vi "Generate Subclasses.vi"(8 "Class Ref Map":T1, 9 "Owning LVLib":refnum<vi>, 10 "Inheritance Map":T1, 11 "Base Class":refnum<vi>) -> (0 "Augmented Class Ref Map":T1, 1 "Owning LVLib Dup":refnum<vi>, 2 "Reduced Inheritance Map":T1, 3 "Base Class Dup":refnum<vi>)   [LabVIEW 2013]
uses:
  <userlib>/ICON Technologies/ICON Maps/lvlib/Map.ctl
  <userlib>/ICON Technologies/ICON Maps/ICON Maps.lvlib
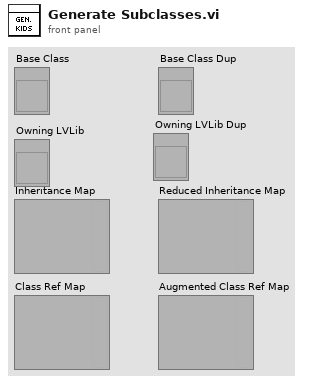
[diagram p1: front panel]
types:
  T1 = typedef "ICON Maps.lvlib/Map.ctl" = variant
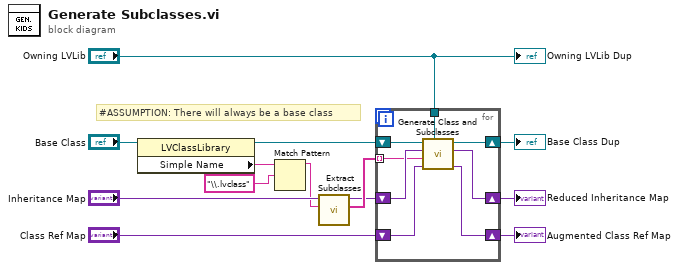
[diagram p0: block diagram]
diagram:
  # "#ASSUMPTION: There will always be a base class"
  n1 = property class="LVClassLibrary"(reference="Base Class") -> (reference out=w4:refnum<vi>, "Simple Name"=w7:string)  [unwired: 1 in, 1 out]
  n2 = Match Pattern(string=w7, regular expression="\\.lvclass") -> (before substring=w6:string)  [unwired: 1 in, 3 out]
  n3 = call "Extract Subclasses.vi"("Base Class Name"=w6, "Inheritance Map"="Inheritance Map") -> ("Subclass Names"=w12:string[], "Reduced Inheritance Map"=w11:T1)  [unwired: 8 in]
  n4 = for {
    tunnel: "Owning LVLib" -> [w21]
    tunnel: w12 -> [w18] mode=indexing
    shift-right: [w20] -> w9
    shift-left: w11 -> [w19]
    shift-right: [w16] -> w13
    shift-left: w4 -> [w17]
    shift-right: [w14] -> w1
    shift-left: "Class Ref Map" -> [w15]
    n5 = call "Generate Class and Subclasses.vi"("Owning LVLib"=w21, "Class Ref Map"=w15, "Class Name"=w18, "Inheritance Map"=w19, "Base Class"=w17) -> ("Augmented Class Ref Map"=w14:T1, "Reduced Inheritance Map"=w20:T1, "Base Class Dup"=w16:refnum<vi>)  [unwired: 4 in]
  }
  "Base Class Dup" <- w13
  "Reduced Inheritance Map" <- w9
  "Augmented Class Ref Map" <- w1
  "Owning LVLib Dup" <- "Owning LVLib"
